vi "test_trace_variables_.vi"() -> ()   [LabVIEW 2013]
panel:
  out "properties":T1
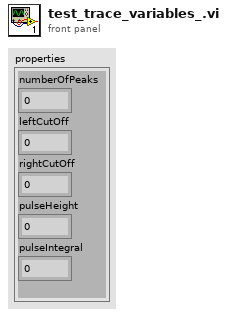
[diagram p1: front panel]
types:
  T1 = cluster{"numberOfPeaks":i16, "leftCutOff":i16, "rightCutOff":i16, "pulseHeight":i16, "pulseIntegral":i32}
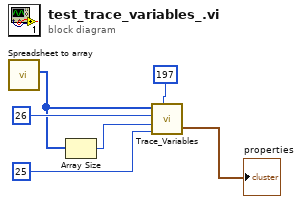
[diagram p0: block diagram]
diagram:
  n1 = call "Spreadsheet to array.vi"() -> ("Array"=w3:u16[])  [unwired: 8 in, 3 out]
  n2 = Array Size(array=w3) -> (size(s)=w4:i32)
  n3 = call "Trace_Variables.vi"("data_12_bit"=w3, "peakThreshold"=u16 26, "traceLength"=w4, "baselineThreshold"=u16 25, "Baseline"=197 ("return type")) -> ("properties"=→"properties":T1)  [unwired: 1 out]
